vi "niLvFpga_WriteBigControl_cRIO-9049.vi"(0 "session in":u32, 7 "Address":u32, 9 "Data In":u32[](array[numeric]), 11 "error in":errorcluster) -> (4 "session out":u32, 15 "error out":errorcluster)   [LabVIEW 2017]
uses:
  NiFpgaLv.dll
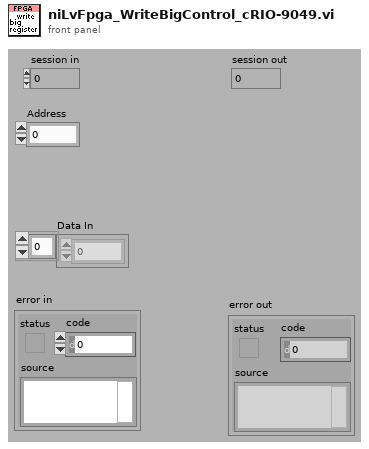
[diagram p1: front panel]
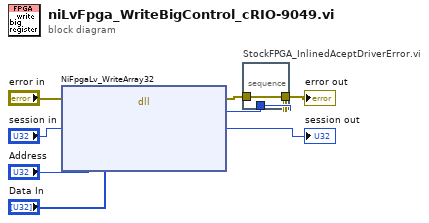
[diagram p0: block diagram]
diagram:
  n1 = dll-call lib="NiFpgaLv.*" fn="NiFpgaLv_WriteArray32" label="niLvFpgaWriteBigControl"(error in="error in", "sessionID"="session in", "offset"="Address", "Data"="Data In") -> (error out=w5:errorcluster, "status"=w3:i32, "sessionID"=→"session out":u32)  [unwired: 4 in, 1 out]
  n2 = stacked-sequence "StockFPGA_InlinedAceptDriverError.vi" {
    tunnel: w5 -> [w9]
    tunnel: w3 -> [w11]
    tunnel: [w10] -> w4
    frame #0 {
      n3 = case shown="Default" w11 {
        selector: w11 -> [_ w13]
        tunnel: [w12 w15] -> w10
        tunnel: w9 -> [w12 w16]
        frame 0 {
        }
        frame Default {
          n4 = Greater Than 0?(x=w13) -> (x > 0?=w14:bool)
          n5 = call <vilib>:"Error Cluster From Error Code.vi"("is warning? (False)"=w14, "error in (no error)"=w16, "error code (0)"=w13) -> ("error out"=w15:errorcluster)  [unwired: 6 in]
        }
      }
    }
  }
  "error out" <- w4
